vi "Stop_Base_Station_Emulator.vi"(8 "error in (no error)":errorcluster, 10 "Cellular Technology":T1, 11 "Base Station":T2) -> (0 "error out":errorcluster, 1 "Output String":string)   [LabVIEW 2021]
uses:
  Controls/Base_Station_Emulator.ctl
  Controls/Cellular_Technology.ctl
  Controls/TCP_FGV.ctl
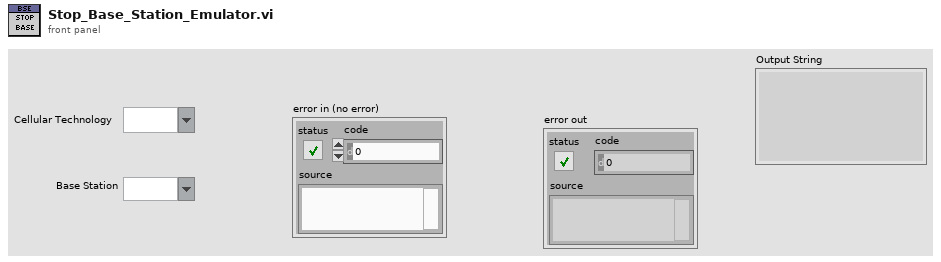
[diagram p1: front panel]
types:
  T1 = typedef "Cellular_Technology.ctl" = string
  T2 = typedef "Base_Station_Emulator.ctl" = string
  T3 = typedef "TCP_FGV.ctl" = enum16{"Open", "Read", "Write", "Close"}
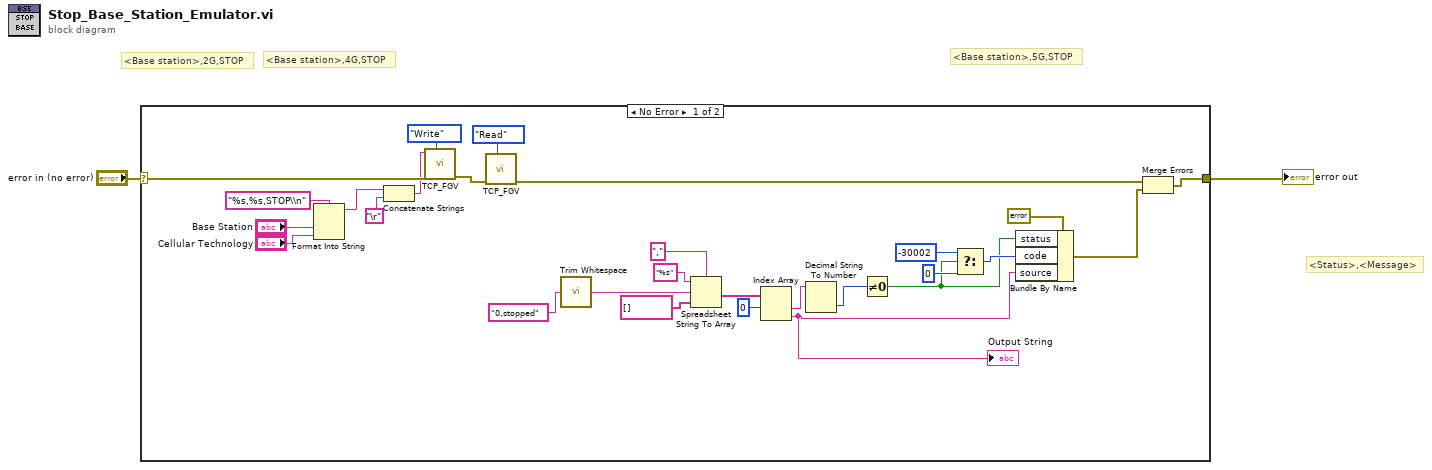
[diagram p0: block diagram]
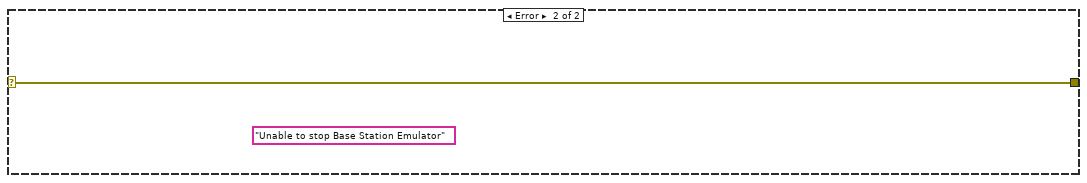
[diagram p2: hidden frame]
diagram:
  # "<Status>,<Message>"
  # "<Base station>,5G,STOP"
  # "<Base station>,4G,STOP"
  # "<Base station>,2G,STOP"
  n1 = case shown="No Error" "error in (no error)" {
    selector: "error in (no error)" -> [w27 w31]
    tunnel: [w6 w31] -> w2
    frame No Error {
      n2 = Format Into String(format string="%s,%s,STOP\\n", "Base Station", "Cellular Technology") -> (resulting string=w25:string)  [unwired: 2 in, 1 out]
      n3 = Concatenate Strings(w25, "\r") -> (w24:string)
      n4 = call "TCP_FGV.vi"("Command"=w24, "error in (no error)"=w27, "Operation"=TCP_FGV."Write") -> ("error out"=w8:errorcluster)  [unwired: 6 in, 1 out]
      n5 = call "TCP_FGV.vi"("error in (no error)"=w8, "Operation"=TCP_FGV."Read") -> ("error out"=w13:errorcluster)  [unwired: 7 in, 1 out]
      n6 = call <vilib>:"Trim Whitespace.vi"("string"="0,stopped" ("Data Out")) -> ("trimmed string"=w22:string)  [unwired: 1 in]
      n7 = Spreadsheet String To Array(delimiter (Tab)=",", format string="%s", spreadsheet string=w22, array type (2D Dbl)=string[] []) -> (array=w21:string[])
      n8 = Index Array(array=w21, index #1=0 ("index")) -> (element #1=w10:string, element #2=w7:string)  [unwired: 1 in]
      "Output String" <- w7
      n9 = Decimal String To Number(string=w10) -> (number=w4:i32)  [unwired: 2 in, 1 out]
      n10 = Not Equal To 0?(x=w4) -> (x != 0?=w9:bool)
      n11 = Select(t=-30002 ("code"), s=w9, f=0 ("code")) -> (s? t:f=w23:i32)
      n12 = Bundle By Name(cluster=errorcluster {"status"=FALSE, "code"=0, "source"=""} ("error constant"), "status"=w9, "code"=w23, "source"=w7) -> (w12:errorcluster)
      n13 = Merge Errors(w13, w12) -> (w6:errorcluster)
    }
    frame Error {
      (unwired) "Unable to stop Base Station Emulator" ("source")
    }
  }
  "error out" <- w2
